vi "Source Names.vi"(4 "Events in":T1[](array[typedef])) -> (6 "Sources":string[](array[string]), 7 "Events":T1[](array[typedef]))   [LabVIEW 2020, in "VolatusGUI.lvlib" / "Event Viewer Module.lvclass"]
uses:
  Event Viewer Module.lvclass
  Event Element.ctl
  Event Viewer Module.lvclass/Event Viewer Module.ctl
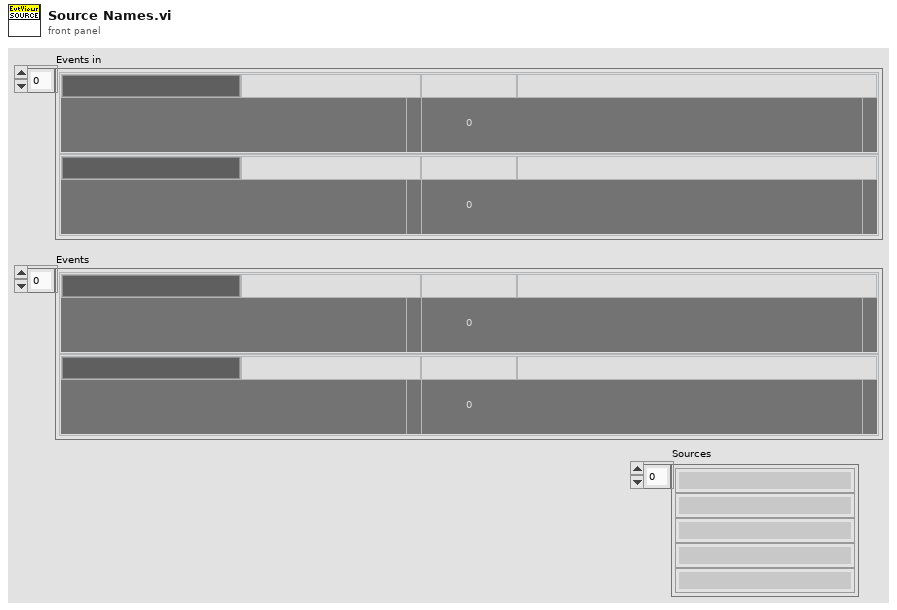
[diagram p1: front panel]
types:
  T1 = typedef "VolatusGUI.lvlib/Event Viewer Module.lvclass/Event Element.ctl" = cluster{"Node":string, "Node Color":u32, "Timestamp":string, "TS Color":u32, "Level":string, "Level Color":u32, "Context":string, "Context Color":u32, "Message":string, "Error Code":i32, "Error Source":string}
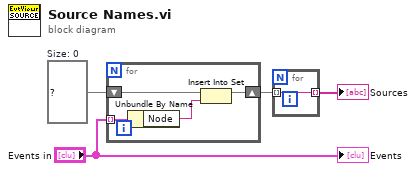
[diagram p0: block diagram]
diagram:
  w3 = set{string} {}  # Size: 0
  n1 = for {
    tunnel: "Events in" -> [w8] mode=indexing
    shift-right: [w5] -> w2
    shift-left: w3 -> [w7]
    n2 = Unbundle By Name(w8) -> ("Node"=w6:string)
    n3 = Insert Into Set(10:w6, 11:w7) -> (3:w5:set{string})  [unwired: 1 out]
  }
  n4 = for {
    tunnel: w2 -> [w9] mode=indexing
    tunnel: [w9] -> w1 mode=indexing
  }
  "Sources" <- w1
  "Events" <- "Events in"
